vi "PrepareFileForLoad.vi"(0 "DIMControSet in":refnum<vi>[](array[refnum]), 1 "SetValueInfo in":refnum<vi>[](array[refnum]), 2 "ListOfBases_Data":refnum<vi>, 3 "Display Message":bool, 4 "Load Value Name Array":string[](array[string]), 5 "Load Value Array":string[](array[string])) -> (15 "Name Array":string[](array[string]), 18 "indexed loaded Array":dbl[][](array[numeric]))   [LabVIEW 2014, in "Panels.lvlib"]
uses:
  Panels.lvlib
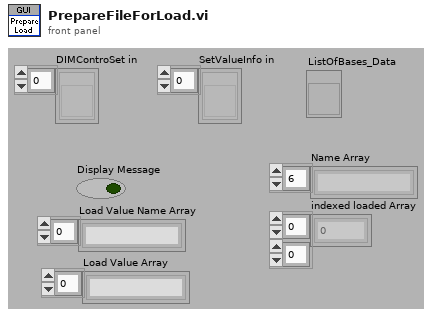
[diagram p1: front panel]
types:
  T1 = cluster{"data":string, "no link":bool, "quality":i32, "timeStamp":dbl}
  T2 = cluster{"data":dbl[], "no link":bool, "quality":i32, "timeStamp":dbl}
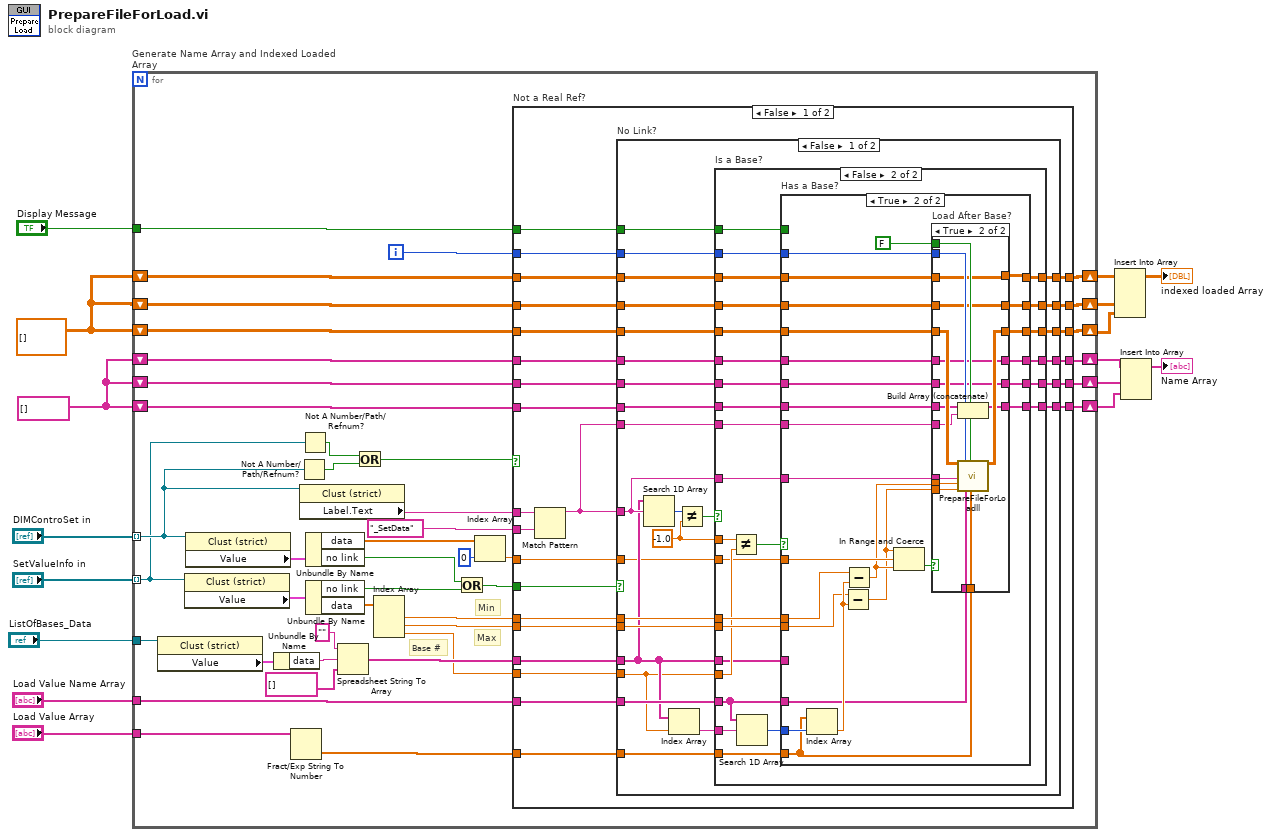
[diagram p0: block diagram]
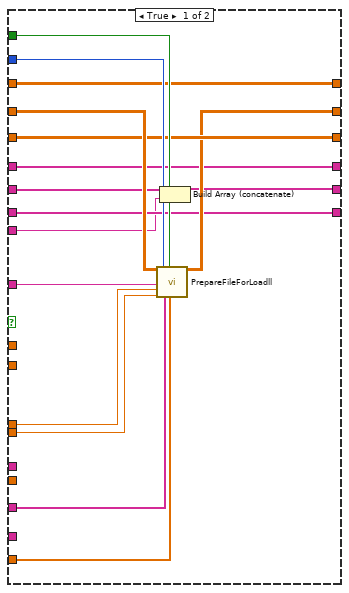
[diagram p2: hidden frame]
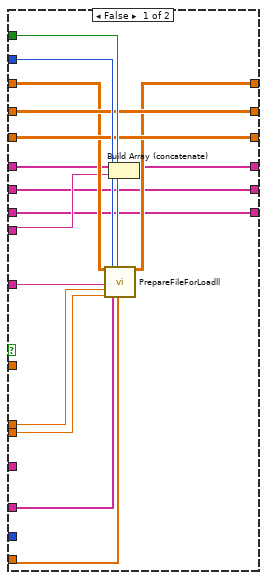
[diagram p3: hidden frame]
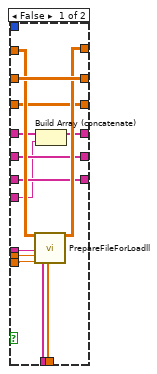
[diagram p4: hidden frame]
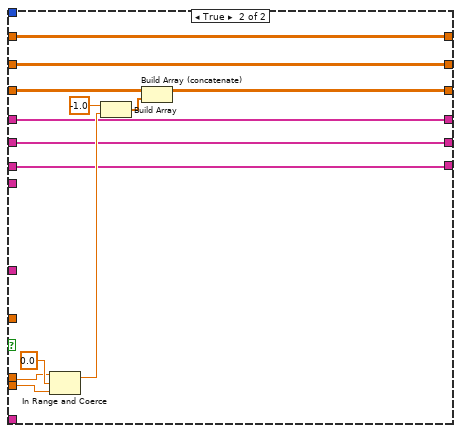
[diagram p5: hidden frame]
diagram:
  w10 = dbl[][] []
  w5 = string[] [] ("array")
  n1 = for "Generate Name Array and Indexed Loaded Array" {
    tunnel: "Load Value Name Array" -> [w44]
    tunnel: "Load Value Array" -> [w58]
    tunnel: "DIMControSet in" -> [w52] mode=indexing
    shift-right: [w17] -> w2
    shift-left: w5 -> [w54]
    tunnel: "Display Message" -> [w53]
    tunnel: "SetValueInfo in" -> [w43] mode=indexing
    shift-right: [w46] -> w6
    shift-left: w10 -> [w47]
    tunnel: "ListOfBases_Data" -> [w38]
    shift-right: [w25] -> w8
    shift-left: w10 -> [w26]
    shift-right: [w27] -> w7
    shift-left: w10 -> [w28]
    shift-right: [w19] -> w4
    shift-left: w5 -> [w20]
    shift-right: [w18] -> w3
    shift-left: w5 -> [w21]
    i -> [w45]
    # "Base #"
    # "Max"
    # "Min"
    n2 = property class="Clust (strict)"(reference=w38) -> ("Value"=w37:T1)  [unwired: 1 in, 2 out]
    n3 = property class="Clust (strict)"(reference=w43) -> ("Value"=w51:T2)  [unwired: 1 in, 2 out]
    n4 = property class="Clust (strict)"(reference=w52) -> ("Value"=w39:T2)  [unwired: 1 in, 2 out]
    n5 = Unbundle By Name(w37) -> ("data"=w35:string)
    n6 = Fract/Exp String To Number(string=w58) -> (number=w57:dbl[])  [unwired: 3 in, 1 out]
    n7 = Not A Number/Path/Refnum?(number/path/refnum=w52) -> (NaN/Path/Refnum?=w41:bool)
    n8 = Not A Number/Path/Refnum?(number/path/refnum=w43) -> (NaN/Path/Refnum?=w42:bool)
    n9 = property class="Clust (strict)"(reference=w52) -> ("Label.Text"=w55:string)  [unwired: 1 in, 2 out]
    n10 = Unbundle By Name(w39) -> ("data"=w24:dbl[], "no link"=w33:bool)
    n11 = Unbundle By Name(w51) -> ("no link"=w32:bool, "data"=w50:dbl[])
    n12 = Spreadsheet String To Array(format string="", spreadsheet string=w35, array type (2D Dbl)=string[] []) -> (array=w30:string[])  [unwired: 1 in]
    n13 = Or(x=w42, y=w41) -> (x .or. y?=w40:bool)
    n14 = Index Array(array=w50) -> (element #1=w49:dbl, element #2=w48:dbl, element #3=w29:dbl)  [unwired: 3 in]
    n15 = Or(x=w33, y=w32) -> (x .or. y?=w31:bool)
    n16 = Index Array(array=w24, index=0) -> (element=w22:dbl)
    n17 = case "Not a Real Ref?" shown="False" w40 {
      tunnel: w44 -> [w76 _]
      tunnel: w57 -> [w75 _]
      tunnel: "_SetData" ("regular expression") -> [w83 _]
      tunnel: w55 -> [w82 _]
      tunnel: w54 -> [w65 w239]
      tunnel: w53 -> [w74 _]
      tunnel: w49 -> [w81 _]
      tunnel: w48 -> [w77 _]
      tunnel: w45 -> [w78 _]
      tunnel: w47 -> [w80 w244]
      tunnel: [w79 w244] -> w46
      tunnel: w31 -> [w73 _]
      tunnel: w30 -> [w72 _]
      tunnel: w29 -> [w71 _]
      tunnel: w28 -> [w70 w243]
      tunnel: [w69 w243] -> w27
      tunnel: w26 -> [w68 w242]
      tunnel: [w67 w242] -> w25
      tunnel: w22 -> [w66 _]
      tunnel: w21 -> [w63 w240]
      tunnel: w20 -> [w64 w241]
      tunnel: [w62 w241] -> w19
      tunnel: [w61 w240] -> w18
      tunnel: [w59 w239] -> w17
      frame False {
        n18 = Match Pattern(string=w82, regular expression=w83) -> (before substring=w60:string)  [unwired: 1 in, 3 out]
        n19 = case "No Link?" shown="False" w73 {
          tunnel: w65 -> [w110 w226]
          tunnel: w60 -> [w101 _]
          tunnel: w81 -> [w105 w231]
          tunnel: w80 -> [w109 w233]
          tunnel: [w108 w232] -> w79
          tunnel: w78 -> [w107 _]
          tunnel: w77 -> [w104 w234]
          tunnel: w76 -> [w103 _]
          tunnel: w75 -> [w102 _]
          tunnel: w74 -> [w106 _]
          tunnel: w72 -> [w93 _]
          tunnel: w71 -> [w92 _]
          tunnel: w70 -> [w97 w230]
          tunnel: [w96 w230] -> w69
          tunnel: w68 -> [w95 w229]
          tunnel: [w94 w229] -> w67
          tunnel: w66 -> [w90 _]
          tunnel: w64 -> [w88 w228]
          tunnel: w63 -> [w89 w227]
          tunnel: [w87 w228] -> w62
          tunnel: [w86 w227] -> w61
          tunnel: w60 -> [w85 _]
          tunnel: [w84 w226] -> w59
          frame False {
            w99 = -1.0 ("y")
            n20 = Search 1D Array(1D array=w93, element=w101) -> (index of element=w100:i32)  [unwired: 1 in]
            n21 = Index Array(array=w93, index=w92) -> (element=w91:string)
            n22 = Not Equal?(x=w100, y=w99) -> (x != y?=w98:bool)
            n23 = case "Is a Base?" shown="False" w98 {
              tunnel: w110 -> [w115 w153]
              tunnel: w109 -> [w118 w152]
              tunnel: [w118 w151] -> w108
              tunnel: w107 -> [w126 w150]
              tunnel: w106 -> [w125 w149]
              tunnel: w105 -> [w124 w148]
              tunnel: w104 -> [w123 w147]
              tunnel: w103 -> [w122 w136]
              tunnel: w102 -> [w121 w146]
              tunnel: w92 -> [_ w144]
              tunnel: w93 -> [_ w143]
              tunnel: w101 -> [w120 w142]
              tunnel: w99 -> [_ w141]
              tunnel: w97 -> [w119 w140]
              tunnel: [w117 w139] -> w96
              tunnel: w95 -> [w116 w138]
              tunnel: [w116 w137] -> w94
              tunnel: w91 -> [_ w135]
              tunnel: w90 -> [_ w133]
              tunnel: w89 -> [w113 w132]
              tunnel: w88 -> [w114 w131]
              tunnel: [w114 w130] -> w87
              tunnel: [w111 w129] -> w86
              tunnel: w85 -> [w112 w128]
              tunnel: [w115 w127] -> w84
              frame True {
                n24 = call "PrepareFileForLoadll.vi"("indexed loaded Array"=w119, "Nickname"=w120, "Min"=w124, "Max"=w123, "Index"=w126, "Load Value Name Array"=w122, "Display Message"=w125, "Load Value Array"=w121) -> ("indexed loaded Array"=w117:dbl[][])  [unwired: 10 in, 1 out]
                n25 = Build Array (concatenate)(w113, w112) -> (w111:string[])
              }
              frame False {
                n26 = Not Equal?(x=w141, y=w144) -> (x != y?=w145:bool)
                n27 = Search 1D Array(1D array=w136, element=w135) -> (index of element=w134:i32)  [unwired: 1 in]
                n28 = case "Has a Base?" shown="True" w145 {
                  tunnel: w153 -> [w154 w189]
                  tunnel: w152 -> [w161 w188]
                  tunnel: [w161 w180] -> w151
                  tunnel: w150 -> [w169 w187]
                  tunnel: w149 -> [w168 _]
                  tunnel: w142 -> [w167 w190]
                  tunnel: w148 -> [w166 w181]
                  tunnel: w147 -> [w165 w182]
                  tunnel: w136 -> [w164 w192]
                  tunnel: w146 -> [w163 w191]
                  tunnel: w143 -> [_ _]
                  tunnel: w140 -> [w162 w185]
                  tunnel: [w162 w184] -> w139
                  tunnel: w138 -> [w160 w178]
                  tunnel: [w159 w179] -> w137
                  tunnel: w134 -> [_ w194]
                  tunnel: w133 -> [_ w183]
                  tunnel: w132 -> [w155 w177]
                  tunnel: w131 -> [w158 w176]
                  tunnel: [w156 w175] -> w130
                  tunnel: [w155 w174] -> w129
                  tunnel: w128 -> [w157 w173]
                  tunnel: [w154 w172] -> w127
                  frame False {
                    n29 = call "PrepareFileForLoadll.vi"("indexed loaded Array"=w160, "Nickname"=w167, "Min"=w166, "Max"=w165, "Index"=w169, "Load Value Name Array"=w164, "Display Message"=w168, "Load Value Array"=w163) -> ("indexed loaded Array"=w159:dbl[][])  [unwired: 10 in, 1 out]
                    n30 = Build Array (concatenate)(w158, w157) -> (w156:string[])
                  }
                  frame True {
                    n31 = Index Array(array=w191, index=w194) -> (element=w195:dbl)
                    n32 = Subtract(x=w182, y=w195) -> (x-y=w170:dbl)
                    n33 = Subtract(x=w181, y=w195) -> (x-y=w171:dbl)
                    n34 = In Range and Coerce(upper limit=w170, x=w183, lower limit=w171) -> (In Range?=w186:bool)  [unwired: 1 out]
                    n35 = case "Load After Base?" shown="True" w186 {
                      tunnel: FALSE ("Display Message") -> [_ w225]
                      tunnel: w192 -> [w205 w224]
                      tunnel: w191 -> [w204 w223]
                      tunnel: w190 -> [w208 w222]
                      tunnel: w189 -> [w200 w212]
                      tunnel: w188 -> [w201 w221]
                      tunnel: w187 -> [_ w220]
                      tunnel: w171 -> [w207 w219]
                      tunnel: w170 -> [w206 w218]
                      tunnel: w185 -> [w209 w217]
                      tunnel: [w209 w217] -> w184
                      tunnel: [w201 w216] -> w180
                      tunnel: [w203 w215] -> w179
                      tunnel: w178 -> [w202 w215]
                      tunnel: w177 -> [w199 w213]
                      tunnel: w176 -> [w198 w214]
                      tunnel: [w197 w214] -> w175
                      tunnel: [w199 w213] -> w174
                      tunnel: w173 -> [w196 w211]
                      tunnel: [w200 w210] -> w172
                      frame False {
                        n36 = call "PrepareFileForLoadll.vi"("indexed loaded Array"=w202, "Nickname"=w208, "Min"=w207, "Max"=w206, "Load Value Name Array"=w205, "Load Value Array"=w204) -> ("indexed loaded Array"=w203:dbl[][])  [unwired: 12 in, 1 out]
                        n37 = Build Array (concatenate)(w198, w196) -> (w197:string[])
                      }
                      frame True {
                        n38 = Build Array (concatenate)(w212, w211) -> (w210:string[])
                        n39 = call "PrepareFileForLoadll.vi"("indexed loaded Array"=w221, "Nickname"=w222, "Min"=w219, "Max"=w218, "Index"=w220, "Load Value Name Array"=w224, "Display Message"=w225, "Load Value Array"=w223) -> ("indexed loaded Array"=w216:dbl[][])  [unwired: 10 in, 1 out]
                      }
                    }
                  }
                }
              }
            }
          }
          frame True {
            n40 = In Range and Coerce(upper limit=w231, x=0.0, lower limit=w234) -> (coerced(x)=w238:dbl)  [unwired: 1 out]
            n41 = Build Array(-1.0 ("element"), w238) -> (w236:dbl[])
            n42 = Build Array (concatenate)(w233, w236) -> (w232:dbl[][])
          }
        }
      }
      frame True {
      }
    }
  }
  n43 = Insert Into Array(array=w8, new element #1=w7, new element #2=w6) -> (→"indexed loaded Array":dbl[][])  [unwired: 2 in]
  n44 = Insert Into Array(array=w4, new element #1=w3, new element #2=w2) -> (→"Name Array":string[])  [unwired: 1 in]
